vi "GetClassInPPL_VisionAnalysis.vi"(10 "FuncName":string, 11 "appended path":path) -> (3 "object":refnum<class>)   [LabVIEW 2019]
uses:
  <vilib>/Utility/LVLibp/NI_PackedLibraryUtility.lvlib
panel:
  out "error out":errorcluster
  out "path":path
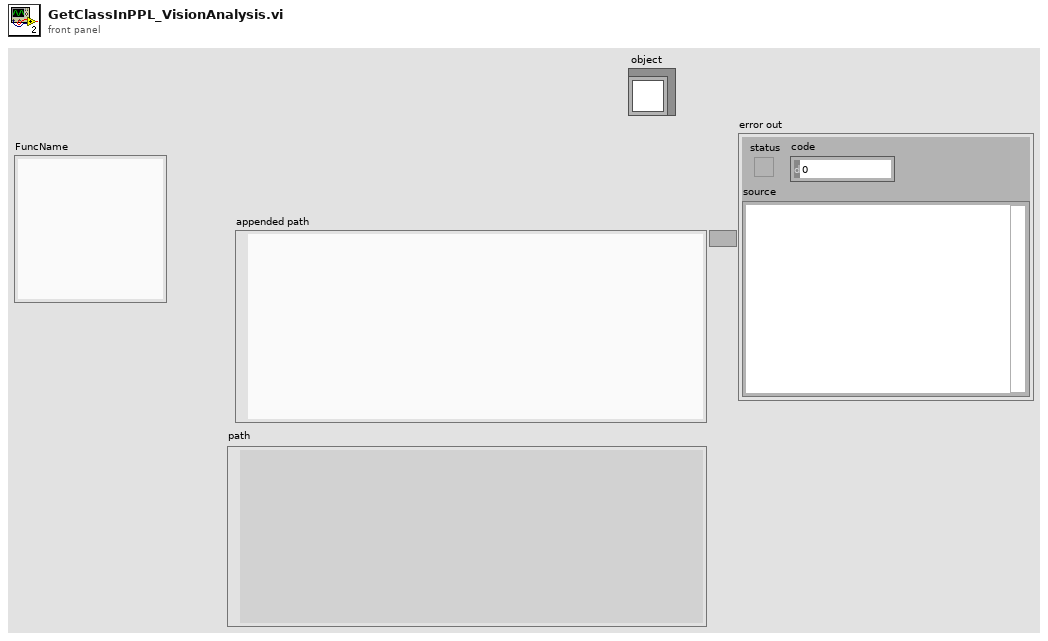
[diagram p1: front panel]
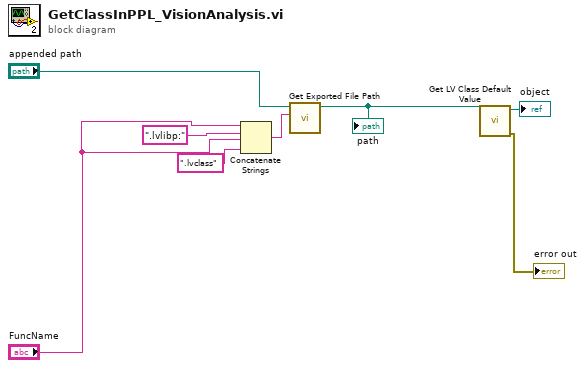
[diagram p0: block diagram]
diagram:
  n1 = Concatenate Strings("FuncName", ".lvlibp:" ("string"), "FuncName", ".lvclass") -> (w8:string)
  n2 = call <vilib>:"Get Exported File Path.vi"("qualified name"=w8, "packed library path"="appended path") -> ("path"=w3:path)  [unwired: 8 in, 1 out]
  "path" <- w3
  n3 = call <vilib>:"Get LV Class Default Value.vi"("class path"=w3) -> ("error out"=→"error out":errorcluster, "object"=→"object":refnum<class>)  [unwired: 9 in]
